vi "read raw tag data.vi"(8 "error in":errorcluster, 11 "engine configuration in":refnum<class "engine configuration.lvclass">) -> (0 "error out":errorcluster, 2 "raw tag data":T1[](array[typedef]), 3 "engine configuration out":refnum<class "engine configuration.lvclass">)   [LabVIEW 2014, in "engine configuration.lvclass"]
doc: "This is intended for \"friends\" but does not use community scoping."
uses:
  engine configuration.lvclass
  Tag Info.ctl
  <vilib>/NI/Tag Bus/tag/tag descriptor.lvclass
  engine configuration.lvclass/engine configuration.ctl
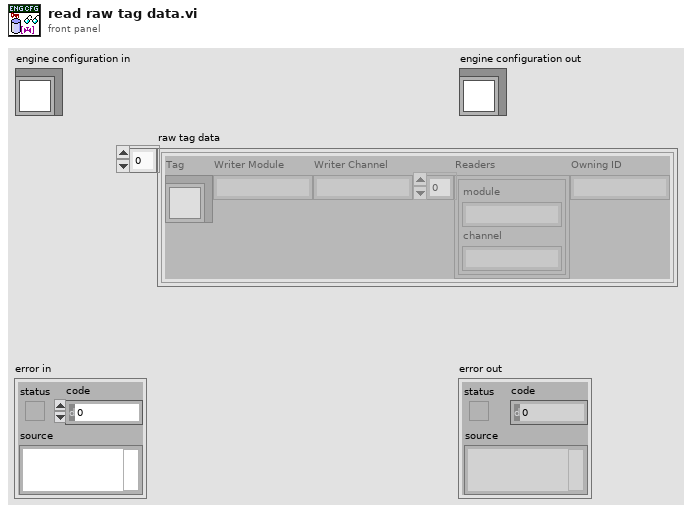
[diagram p1: front panel]
types:
  T1 = typedef "engine configuration.lvclass/Tag Info.ctl" = cluster{"Tag":refnum<class "tag descriptor.lvclass">, "Writer Module":string, "Writer Channel":string, "Readers":cluster{"module":string, "channel":string}[], "Owning ID":string}
  T2 = typedef "engine configuration.lvclass/module channel pairings.ctl" = cluster{"modules":string[], "channels":string[]}
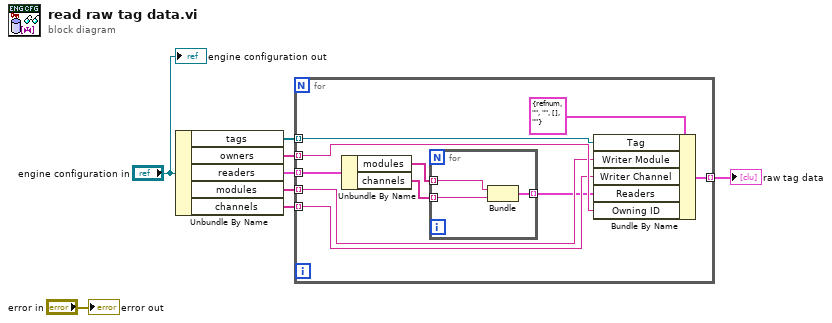
[diagram p0: block diagram]
diagram:
  n1 = Unbundle By Name("engine configuration in") -> ("tags"=w5:refnum<class "tag descriptor.lvclass">[], "owners"=w4:string[], "readers"=w1:T2[], "modules"=w3:string[], "channels"=w2:string[])
  n2 = for {
    tunnel: [w17] -> w6 mode=indexing
    tunnel: w5 -> [w16] mode=indexing
    tunnel: w4 -> [w15] mode=indexing
    tunnel: w3 -> [w14] mode=indexing
    tunnel: w2 -> [w13] mode=indexing
    tunnel: w1 -> [w12] mode=indexing
    n3 = Unbundle By Name(w12) -> ("modules"=w11:string[], "channels"=w10:string[])
    n4 = for {
      tunnel: w11 -> [w21] mode=indexing
      tunnel: w10 -> [w20] mode=indexing
      tunnel: [w19] -> w9 mode=indexing
      n5 = Bundle("String"=w21, "String"=w20) -> (w19:cluster{"String":string, "String":string})  [unwired: 1 in]
    }
    n6 = Bundle By Name(cluster=T1 {"Tag"=refnum, "Writer Module"="", "Writer Channel"="", "Readers"=[], "Owning ID"=""} ("Tag Info"), "Tag"=w16, "Writer Module"=w14, "Writer Channel"=w13, "Readers"=w9, "Owning ID"=w15) -> (w17:T1)
  }
  "raw tag data" <- w6
  "error out" <- "error in"
  "engine configuration out" <- "engine configuration in"
